vi "map_coordinates_xi_fourtyfive_old.vi"(4 "Center Y":dbl, 5 "phi_in":dbl, 6 "Center X":dbl, 7 "a":dbl, 8 "Beta":dbl, 9 "D":dbl, 10 "c":dbl, 11 "b":dbl) -> (2 "b_pixel":dbl, 3 "a_pixel":dbl)   [LabVIEW 2019]
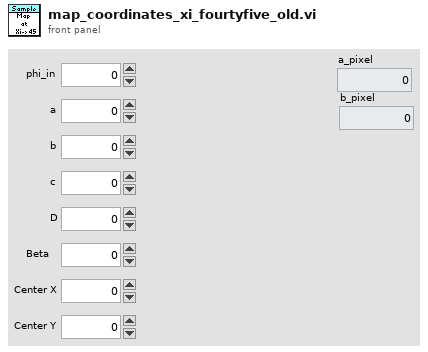
[diagram p1: front panel]
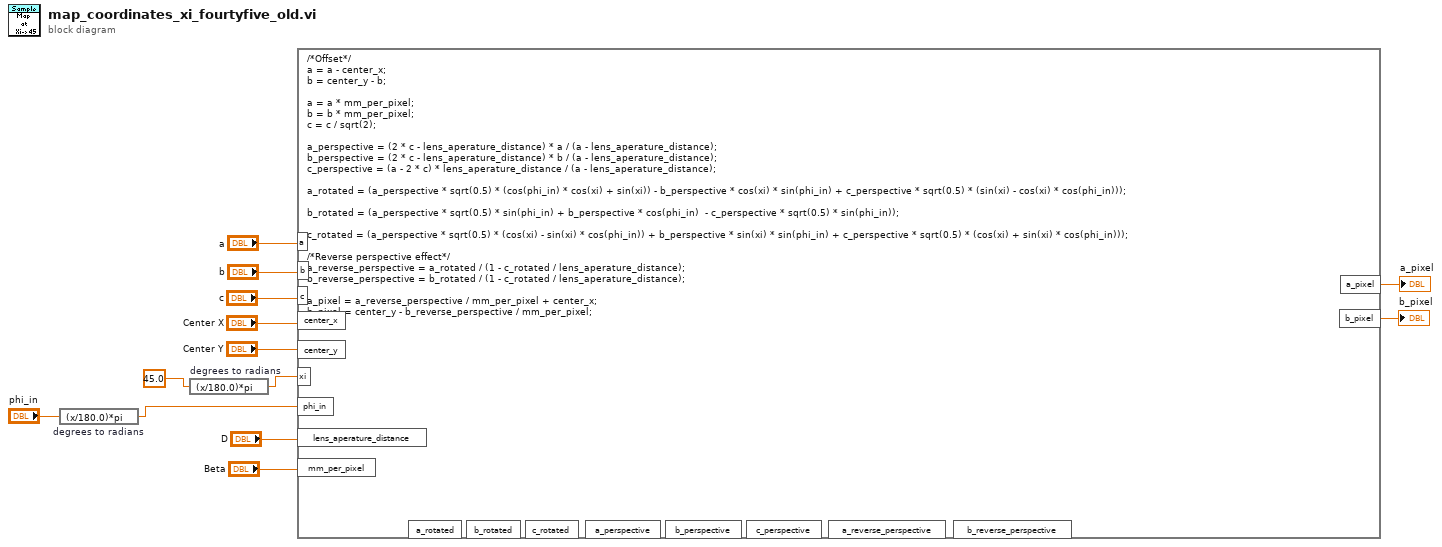
[diagram p0: block diagram]
diagram:
  n1 = expression code="(x/180.0)*pi" "degrees to radians"("phi_in") -> (w5:dbl)
  n2 = expression code="(x/180.0)*pi" "degrees to radians"(45.0 ("input variable")) -> (w2:dbl)
  n3 = formula code="/*Offset*/\na = a - center_x;\nb = center_y - b;\n    \na = a * mm_per_pixel;\nb = b * mm_per_pixel;\nc = c / sqrt(2);\n    \na_perspective = (2 * c - lens_aperature_distance) * a / (a - lens_aperature_distance);\nb_perspective = (2 * c - lens_aperature_distance) * b / (a - lens_aperature_distance);\nc_perspective = (a - 2 * c) * lens_aperature_distance / (a - lens_aperature_distance);\n    \na_rotated = (a_perspective * sqrt(0.5) * (cos(phi_in) * cos(xi) + sin(xi)) - b_perspective * cos(xi) * sin(phi_in) + c_perspective * sqrt(0.5) * (sin(xi) - cos(xi) * cos(phi_in)));\n    \nb_rotated = (a_perspective * sqrt(0.5) * sin(phi_in) + b_perspective * cos(phi_in)  - c_perspective * sqrt(0.5) * sin(phi_in));\n    \nc_rotated = (a_perspective * sqrt(0.5) * (cos(xi) - sin(xi) * cos(phi_in)) + b_perspective * sin(xi) * sin(phi_in) + c_perspective * sqrt(0.5) * (cos(xi) + sin(xi) * cos(phi_in)));\n\n/*Reverse perspective effect*/\na_reverse_perspective = a_rotated / (1 - c_rotated / lens_aperature_distance);\nb_reverse_perspective = b_rotated / (1 - c_rotated / lens_aperature_distance);\n    \na_pixel = a_reverse_perspective / mm_per_pixel + center_x;\nb_pixel = center_y - b_reverse_perspective / mm_per_pixel;"("a"="a", "b"="b", "c"="c", "center_x"="Center X", "center_y"="Center Y", "xi"=w2, "phi_in"=w5, "lens_aperature_distance"="D", "mm_per_pixel"="Beta") -> ("a_pixel"=→"a_pixel":dbl, "b_pixel"=→"b_pixel":dbl)  [unwired: 8 out]
